vi "Create Symbolic Path to Public Documents.vi"() -> ()   [LabVIEW 2018]
doc: "This VI shows how to link the Dashboard to a ONE location in the repo"
panel:
  in  "Close":bool
  # "Instructions to link the Dashboard to a single location:\n\n1. Download and install the Link Shell Extension\n   http://schinagl.priv.at/nt/hardlinkshellext/linkshellextension.html \n2. Delete the FRC Dashboard folder inside C:\\Program Files (x86)\n3. Create a Link between the Build and the C:\\Program Files (x86) folder"
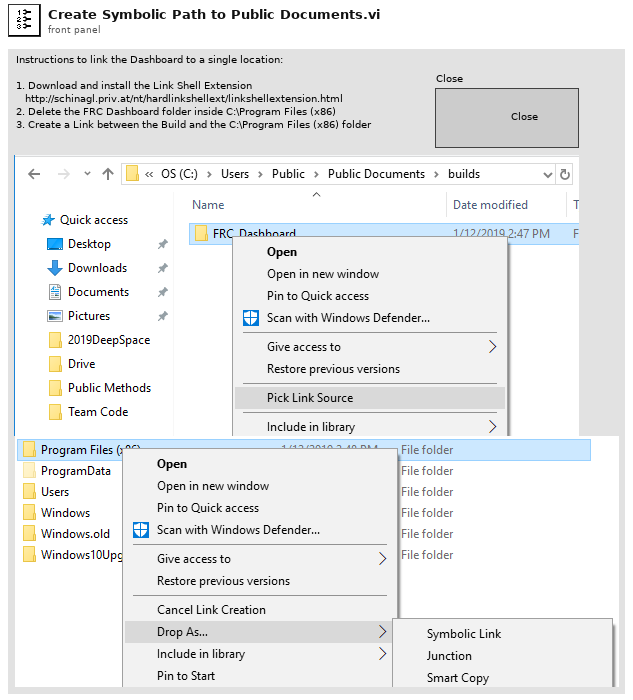
[diagram p1: front panel]
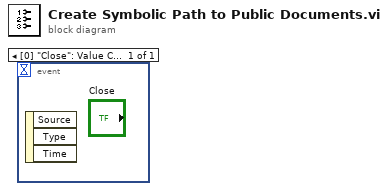
[diagram p0: block diagram]
diagram:
  n1 = event shown="[0] \"Close\": Value Change;  Panel Close" {
    selector: _ -> [_]
    dyn-events: _ -> [_]
    timeout: _ -> [_]
    event "Close": Value Change; Panel Close {
      n2 = event-data() -> ()  [unwired: 1 in, 3 out]
    }
  }
